vi "ThrottleToTorque.vi"(10 "Coeffecients":cluster{"X3":dbl, "X2":dbl, "X1":dbl, "C":dbl}={"X3"=-2.3e-06, "X2"=-0.00383, "X1"=-0.639, "C"=49.9}, 11 "Throttle":dbl=500.0) -> (2 "Newtons":dbl, 3 "Torque":dbl=-1514.6)   [LabVIEW 2011]
doc: "This VI Converts a throttle to a thrust in accordance with the coefficients given. The coefficients should correspond to those of a third order equation that maps the throttle values, to the acceleration the propellor actually generates."
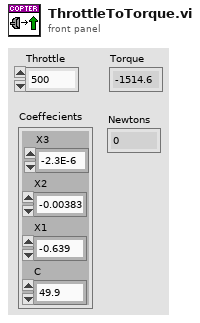
[diagram p1: front panel]
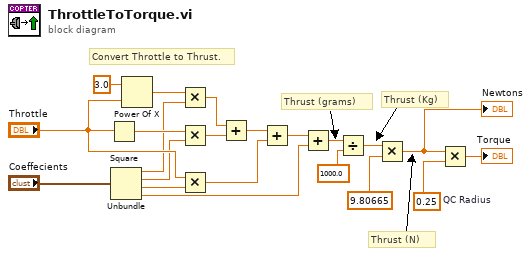
[diagram p0: block diagram]
diagram:
  w3 = 0.25  # QC Radius
  # "Convert Throttle to Thrust."
  # "Thrust (N)"
  # "Thrust (Kg)"
  # "Thrust (grams)"
  n1 = Square(x="Throttle") -> (x^2=w17:dbl)
  n2 = Unbundle("Coeffecients") -> ("X3"=w11:dbl, "X2"=w10:dbl, "X1"=w9:dbl, "C"=w8:dbl)
  n3 = Power Of X(1:"Throttle", 2:3.0 ("y")) -> (0:w15:dbl)
  n4 = Multiply(x=w15, y=w11) -> (x*y=w16:dbl)
  n5 = Multiply(x=w17, y=w10) -> (x*y=w18:dbl)
  n6 = Multiply(x="Throttle", y=w9) -> (x*y=w21:dbl)
  n7 = Add(x=w16, y=w18) -> (x+y=w20:dbl)
  n8 = Add(x=w20, y=w21) -> (x+y=w13:dbl)
  n9 = Add(x=w13, y=w8) -> (x+y=w7:dbl)
  n10 = Divide(x=w7, y=1000.0) -> (x/y=w5:dbl)
  n11 = Multiply(x=w5, y=9.80665) -> (x*y=w1:dbl)
  "Newtons" <- w1
  n12 = Multiply(x=w1, y=w3) -> (x*y=→"Torque":dbl)
